vi "Popup Dispatcher.vi"(6 "Panel":refnum<class "Panel.lvclass">, 8 "error in (no error)":errorcluster, 9 "Popup Return Data":refnum<user-event>, 10 "String in":string, 11 "Generic Data Type in":refnum<class "Generic Data Type.lvclass">) -> (0 "error out":errorcluster, 3 "Generic Data Type out":refnum<class "Generic Data Type.lvclass">)   [LabVIEW 2018, in "Generic Data Type.lvclass"]
uses:
  Generic Data Type.lvclass
  <vilib>/MGI/Panel Manager/Panel/Panel/Panel.lvclass
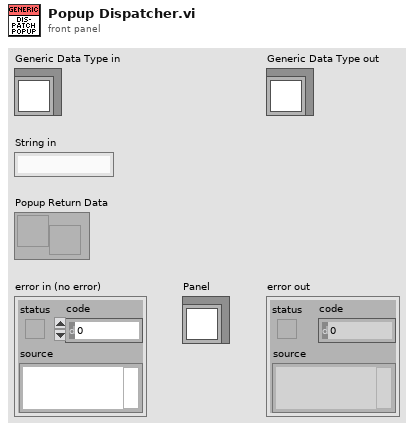
[diagram p1: front panel]
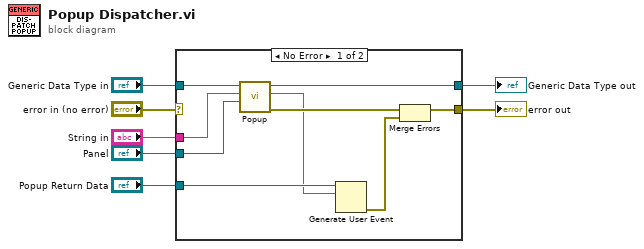
[diagram p0: block diagram]
diagram:
  n1 = case shown="No Error" "error in (no error)" {
    selector: "error in (no error)" -> [_ w18]
    tunnel: [w11 w18] -> w6
    tunnel: [w16 w17] -> w4
    tunnel: "Generic Data Type in" -> [w9 w17]
    tunnel: "String in" -> [w15 _]
    tunnel: "Popup Return Data" -> [w13 _]
    tunnel: "Panel" -> [w8 _]
    frame No Error {
      n2 = call-dynamic "Popup.vi"("Panel"=w8, "String in"=w15, "Generic Data Type in"=w9) -> ("error out"=w14:errorcluster, "String out"=w12:string, "Generic Data Type out"=w16:refnum<class "Generic Data Type.lvclass">)  [unwired: 6 in]
      n3 = Generate User Event(user event=w13, event data cluster=w12) -> (error out=w10:errorcluster)  [unwired: 2 in, 1 out]
      n4 = Merge Errors(w14, w10) -> (w11:errorcluster)
    }
    frame Error {
    }
  }
  "error out" <- w6
  "Generic Data Type out" <- w4
